vi "Get Diagnostics.vi"(8 "error in (no error)":errorcluster, 11 "Instrument Actor in":refnum<class "Instrument Actor.lvclass">) -> (0 "error out":errorcluster, 2 "Diagnostics":string, 3 "Instrument Actor out":refnum<class "Instrument Actor.lvclass">)   [LabVIEW 2024, in "Instrument Actor.lvclass"]
uses:
  Instrument Actor.lvclass
  Instrument Actor.lvclass/Instrument Actor.ctl
  Read Instrument driver.vi
  Write Instrument driver.vi
  NHMFL_Core/Libraries/Instruments/Instrument Driver/Instrument Driver.lvclass
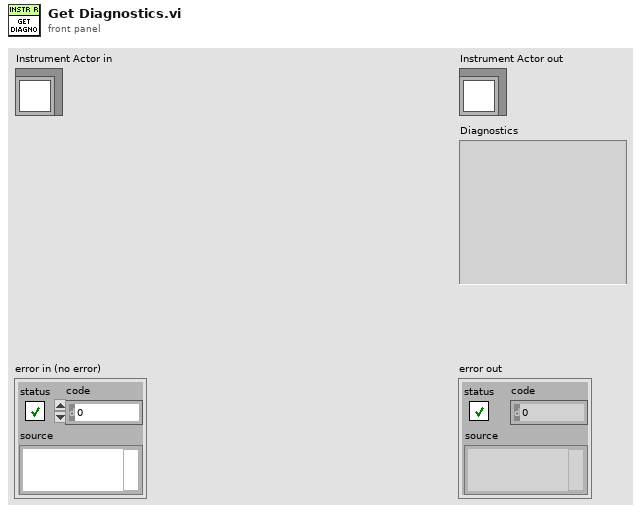
[diagram p1: front panel]
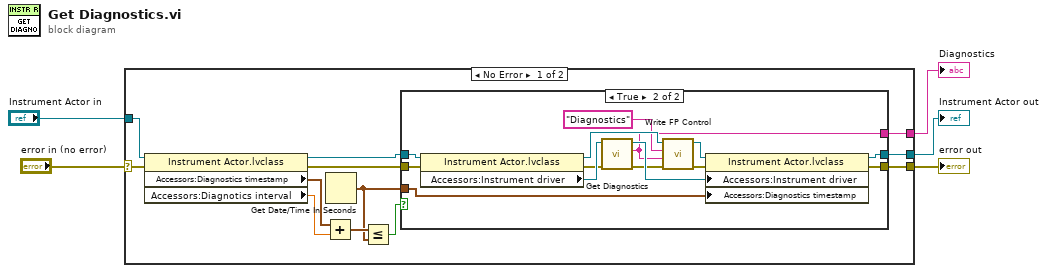
[diagram p0: block diagram]
diagram:
  n1 = case shown="No Error" "error in (no error)" {
    selector: "error in (no error)" -> [w17 w35]
    tunnel: [w6 w35] -> w4
    tunnel: [w7 w34] -> w2
    tunnel: "Instrument Actor in" -> [w16 w34]
    tunnel: [w14 _] -> w1
    frame No Error {
      n2 = property class="Instrument Actor.lvclass"(reference=w16, error in=w17) -> (reference out=w8:refnum<class "Instrument Actor.lvclass">, error out=w15:errorcluster, "Accessors:Diagnostics timestamp"=w10:timestamp, "Accessors:Diagnotics interval"=w12:dbl)
      n3 = Add(x=w10, y=w12) -> (x+y=w13:timestamp)
      n4 = Get Date/Time In Seconds() -> (seconds since 1Jan1904=w9:timestamp)
      n5 = Less Or Equal?(x=w13, y=w9) -> (x <= y?=w11:bool)
      n6 = case shown="True" w11 {
        tunnel: w15 -> [w18 w21]
        tunnel: [_ w22] -> w14
        tunnel: w9 -> [_ w29]
        tunnel: w8 -> [w19 w33]
        tunnel: [w19 w28] -> w7
        tunnel: [w18 w27] -> w6
        frame False {
        }
        frame True {
          n7 = property class="Instrument Actor.lvclass"(reference=w33, error in=w21) -> (reference out=w24:refnum<class "Instrument Actor.lvclass">, error out=w20:errorcluster, "Accessors:Instrument driver"=w32:refnum<class "Instrument Driver.lvclass">)
          n8 = call-dynamic "Get Diagnostics.vi"("error in (no error)"=w20, "Instrument Driver in"=w32) -> ("error out"=w26:errorcluster, "Diagnostics"=w22:string, "Instrument Driver out"=w30:refnum<class "Instrument Driver.lvclass">)  [unwired: 7 in]
          n9 = call-dynamic "Write FP Control.vi"("error in (no error)"=w26, "Control Value"=w22, "Control Name"="Diagnostics", "Measure Object in"=w24) -> ("error out"=w25:errorcluster, "Measure Object out"=w31:refnum<class "Instrument Actor.lvclass">)  [unwired: 6 in]
          n10 = property class="Instrument Actor.lvclass"(reference=w31, error in=w25, "Accessors:Instrument driver"=w30, "Accessors:Diagnostics timestamp"=w29) -> (reference out=w28:refnum<class "Instrument Actor.lvclass">, error out=w27:errorcluster)
        }
      }
    }
    frame Error {
    }
  }
  "error out" <- w4
  "Instrument Actor out" <- w2
  "Diagnostics" <- w1
